vi "example_ping_demo.vi"() -> ()   [LabVIEW 2013]
doc: "This example performs a series of pings to 127.0.0.1 to demonstrate the asynchronous StdOut updates.\n\nThere is a ~1sec delay between pings, so the total execution time should be about 5 seconds, but you can see the StdOut messages as they are\ngenerated, as opposed to waiting for the entire operation to complete.\n\nThe ping command is followed by an \"exit\" command, which fires the \"Process Exited\" event and stops this VI."
uses:
  dotnet_system_exec/dotnet_system_exec.lvclass
panel:
  out "StdErr":string
  out "StdOut":string
  # "This example performs a series of pings to 127.0.0.1 to demonstrate the asynchronous StdOut updates.\n\nThere is a ~1sec delay between pings, so the total execution time should be about 5 seconds, but you can see the StdOut messages as they are\ngenerated, as opposed to waiting for the entire operation to complete.\n\nThe ping command is followed by an \"exit\" command, which fires the \"Process Exited\" event and stops this VI."
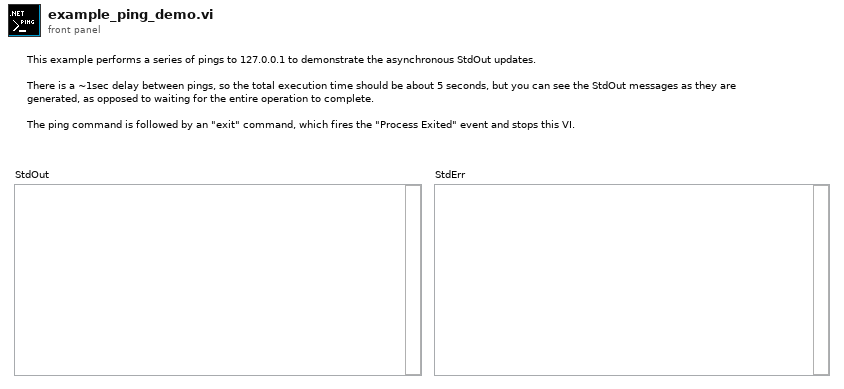
[diagram p1: front panel]
types:
  T1 = cluster{"stdout event":refnum<user-event>, "stderr event":refnum<user-event>, "process_exit event":refnum<user-event>}
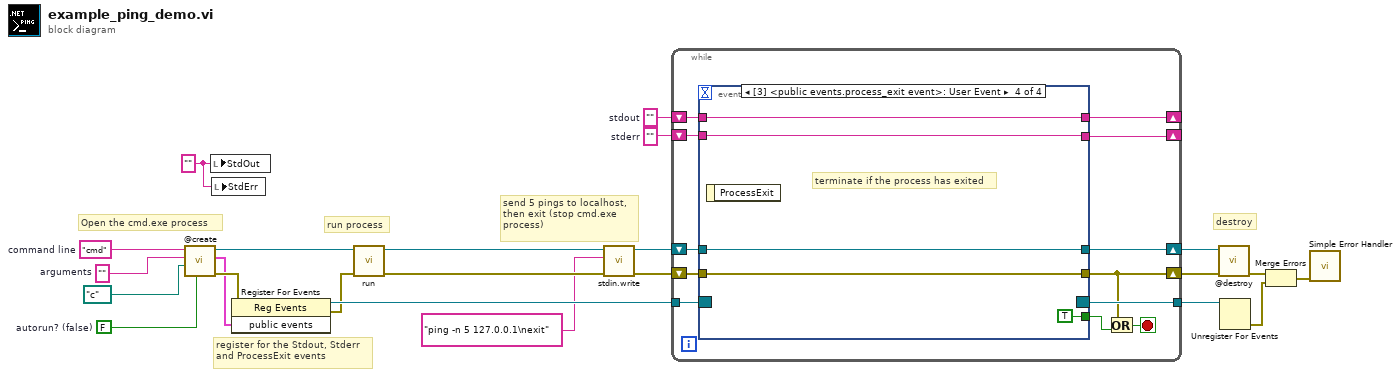
[diagram p0: block diagram]
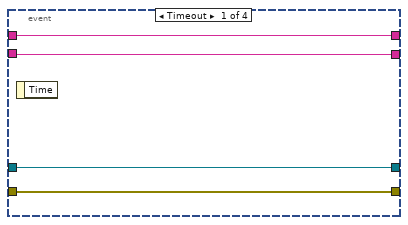
[diagram p2: hidden frame]
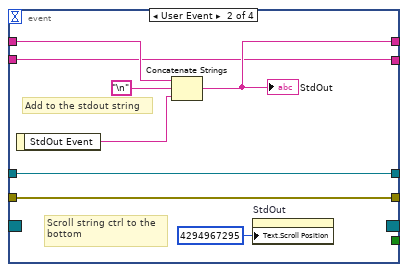
[diagram p3: hidden frame]
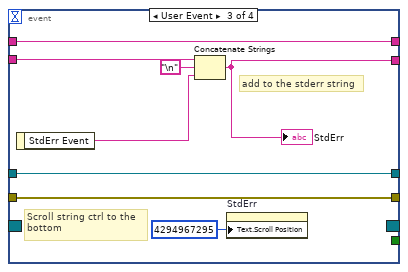
[diagram p4: hidden frame]
diagram:
  w6 = FALSE  # autorun? (false)
  w7 = "" ("Process File Name")
  w9 = ""  # stderr
  w13 = ""  # arguments
  w14 = ""  # stdout
  w15 = "cmd"  # command line
  # "send 5 pings to localhost,\nthen exit (stop cmd.exe \nprocess)"
  # "destroy"
  # "register for the Stdout, Stderr \nand ProcessExit events"
  # "run process"
  # "Open the cmd.exe process"
  n1 = call "@create.vi"("autorun? (false)"=w6, "working directory (c:\\)"=path "c:/" ("working directory"), "arguments (\"\")"=w13, "command line (cmd.exe)"=w15) -> ("error out"=w12:errorcluster, "public events"=w10:T1, "dotnet_system_exec out"=w22:refnum<class "dotnet_system_exec.lvclass">)  [unwired: 5 in]
  n2 = local write "StdOut"(w7) -> ()
  n3 = local write "StdErr"(w7) -> ()
  n4 = register-events(error in=w12, w10) -> (reference out=w21:refnum<event-registration>, error out=w11:errorcluster)  [unwired: 1 in]
  n5 = call "run.vi"("error in (no error)"=w11, "dotnet_system_exec in"=w22) -> ("error out"=w4:errorcluster, "dotnet_system_exec out"=w5:refnum<class "dotnet_system_exec.lvclass">)  [unwired: 8 in]
  n6 = call-dynamic "stdin.write.vi"("error in (no error)"=w4, "stdin"="ping -n 5 127.0.0.1\nexit", "dotnet_system_exec in"=w5) -> ("error out"=w2:errorcluster, "dotnet_system_exec out"=w3:refnum<class "dotnet_system_exec.lvclass">)  [unwired: 7 in]
  n7 = while {
    shift-right: [w35] -> w23
    shift-left: w3 -> [w34]
    shift-right: [w25] -> w19
    shift-left: w2 -> [w33]
    tunnel: w21 -> [w32]
    tunnel: [w31] -> w20
    shift-right: [w29] -> _
    shift-left: w14 -> [w30]
    shift-right: [w27] -> _
    shift-left: w9 -> [w28]
    stop <- w24 stop-if-true
    n8 = event shown="[3] <public events.process_exit event>: User Event" {
      selector: w32 -> [_ _ _ _]
      dyn-events: [_ _ _ _] -> w31
      timeout: _ -> [_ _ _ _]
      tunnel: [w39 w47 w55 w58] -> w35
      tunnel: w34 -> [w39 w47 w55 w58]
      tunnel: w33 -> [w38 w46 w54 w57]
      tunnel: [w38 w46 w54 w57] -> w25
      tunnel: w30 -> [w37 w43 w50 w59]
      tunnel: [w37 w44 w50 w59] -> w29
      tunnel: [_ _ _ TRUE ("ProcessExit")] -> w26
      tunnel: w28 -> [w36 w41 w51 w60]
      tunnel: [w36 w41 w49 w60] -> w27
      event Timeout {
        n9 = event-data() -> ()  [unwired: 1 in, 1 out]
      }
      event User Event {
        # "Scroll string ctrl to the \nbottom"
        # "Add to the stdout string"
        n10 = event-data() -> ("StdOut Event"=w42:string)  [unwired: 1 in]
        n11 = Concatenate Strings(w43, "\n", w42) -> (w44:string)
        "StdOut" <- w44
        n12 = property on="StdOut" class="Str"("Text.Scroll Position"=u32 4294967295) -> ()  [unwired: 2 in, 2 out]
      }
      event User Event {
        # "Scroll string ctrl to the \nbottom"
        # "add to the stderr string"
        n13 = event-data() -> ("StdErr Event"=w52:string)  [unwired: 1 in]
        n14 = Concatenate Strings(w51, "\n", w52) -> (w49:string)
        "StdErr" <- w49
        n15 = property on="StdErr" class="Str"("Text.Scroll Position"=u32 4294967295) -> ()  [unwired: 2 in, 2 out]
      }
      event User Event {
        # "terminate if the process has exited"
        n16 = event-data() -> ()  [unwired: 1 in, 1 out]
      }
    }
    n17 = Or(x=w25, y=w26) -> (x .or. y?=w24:bool)
  }
  n18 = call-dynamic "@destroy.vi"("error in (no error)"=w19, "dotnet_system_exec in"=w23) -> ("error out"=w18:errorcluster)  [unwired: 8 in, 1 out]
  n19 = Unregister For Events(event registration refnum=w20) -> (error out=w17:errorcluster)  [unwired: 1 in]
  n20 = Merge Errors(w18, w17) -> (w16:errorcluster)
  n21 = call <vilib>:"Simple Error Handler.vi"("error in (no error)"=w16) -> ()  [unwired: 4 in, 5 out]
